vi "tsapp_configure_baudrate_can_win32.vi"(1 "AppName":string, 2 "配置波特率":T1={"硬件类型"=3, "硬件子类型"=5, "ABaudrateKbps"=500.0, "AListenOnly"=enum."Normal", "Int120Ohm"=enum."Disable", "EnableChannel"=enum."Enable", "AHwChannel"=0, "AAppChannel"=0} {"AAppChannel" items=["CHN1", "CHN2", "CHN3", "CHN4", "CHN5", "CHN6", "CHN7", "CHN8", "CHN9", "CHN10", "CHN11", "CHN12", "CHN13", "CHN14", "CHN15", "CHN16", "CHN17", "CHN18", "CHN19", "CHN20", "CHN21", "CHN22", "CHN23", "CHN24", "CHN25", "CHN26", "CHN27", "CHN28", "CHN29", "CHN30", "CHN31", "CHN32"]; "AHwChannel" items=["CHN1", "CHN2", "CHN3", "CHN4", "CHN5", "CHN6", "CHN7", "CHN8", "CHN9", "CHN10", "CHN11", "CHN12", "CHN13", "CHN14", "CHN15", "CHN16", "CHN17", "CHN18", "CHN19", "CHN20", "CHN21", "CHN22", "CHN23", "CHN24", "CHN25", "CHN26", "CHN27", "CHN28", "CHN29", "CHN30", "CHN31", "CHN32"]; "硬件子类型" items=["BUS_UNKNOWN_TYPE", "TSCAN_PRO_4", "TSCAN_LITE_2", "TSCANMini", "TSLinMini", "TSCANFDmini", "TSCAN_LIN_IO_2", "TSCAN_LITE_2", "TSCANLIN", "TSCAN_FD_Mini_1"]; "硬件类型" items=["BUS_UNKNOWN_TYPE", "TS_TCP_DEVICE", "XL_USB_DEVICE", "TS_USB_DEVICE", "PEAK_USB_DEVICE", "KVASER_USB_DEVICE", "ZLG_USB_DEVICE", "ICS_USB_DEVICE", "TS_TC1005_DEVICE"]}, 3 "错误输入（无错误）":errorcluster) -> (9 "InitSts":bool, 10 "错误输出":errorcluster)   [LabVIEW 2016]
uses:
  Ctrl/CAN_BaudInfo.ctl
  TSMaster.dll
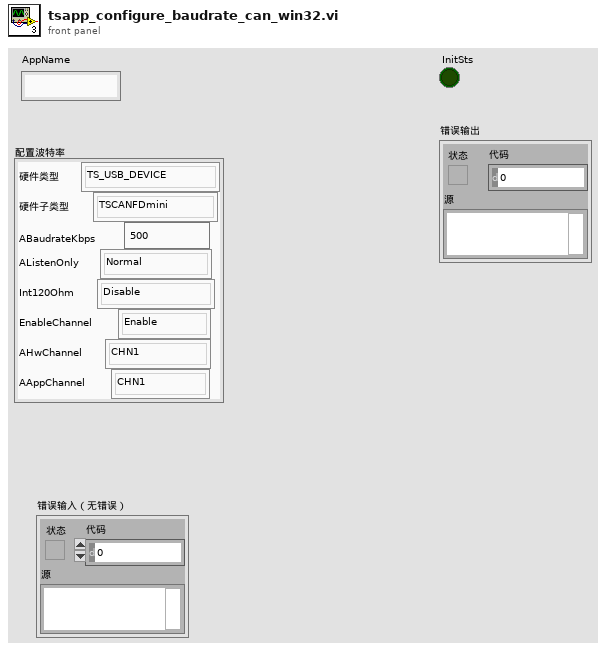
[diagram p1: front panel]
types:
  T1 = typedef "CAN_BaudInfo.ctl" = cluster{"硬件类型":i32, "硬件子类型":i32, "ABaudrateKbps":sgl, "AListenOnly":enum16{"Normal", "ListenOnly"}, "Int120Ohm":enum16{"Disable", "Enable"}, "EnableChannel":enum16{"Disable", "Enable"}, "AHwChannel":i32, "AAppChannel":i32}
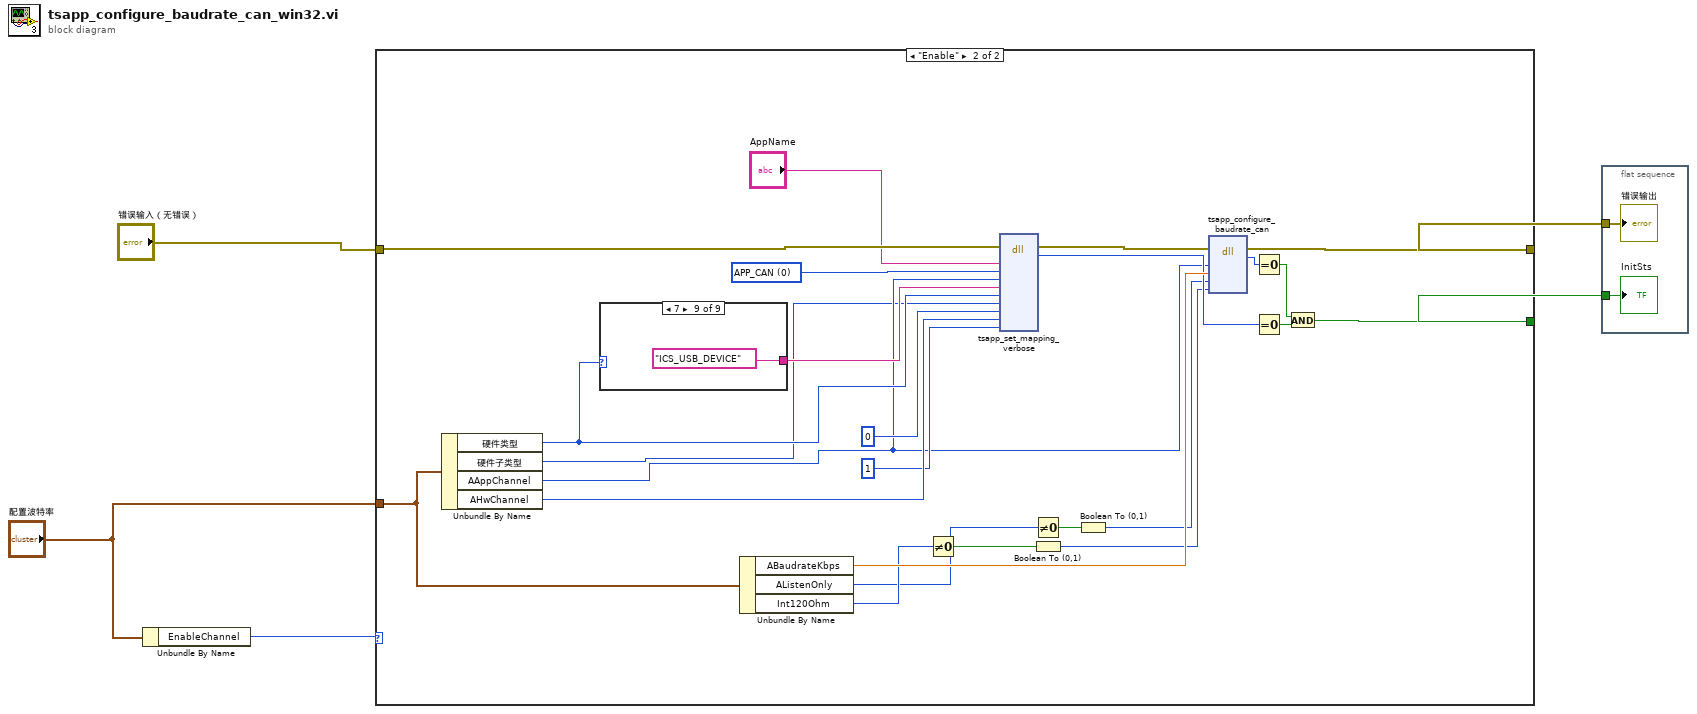
[diagram p0: block diagram]
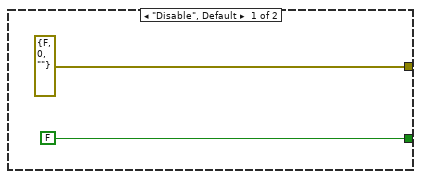
[diagram p2: hidden frame]
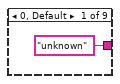
[diagram p3: hidden frame]
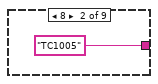
[diagram p4: hidden frame]
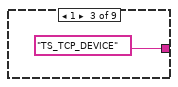
[diagram p5: hidden frame]
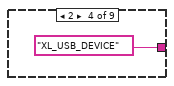
[diagram p6: hidden frame]
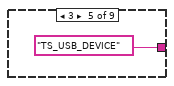
[diagram p7: hidden frame]
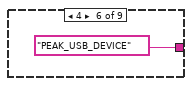
[diagram p8: hidden frame]
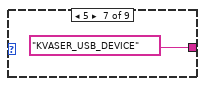
[diagram p9: hidden frame]
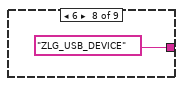
[diagram p10: hidden frame]
diagram:
  n1 = Unbundle By Name("配置波特率") -> ("EnableChannel"=w2:enum16{"Disable", "Enable"})
  n2 = case shown="\"Enable\"" w2 {
    tunnel: "错误输入（无错误）" -> [_ w31]
    tunnel: [errorcluster {"status"=FALSE, "code"=0, "source"=""} ("错误输出") w27] -> w4
    tunnel: [FALSE w14] -> w3
    tunnel: "配置波特率" -> [_ w20]
    frame "Disable", Default {
    }
    frame "Enable" {
      w30 = 0 items=["APP_CAN", "APP_LIN"] ("AAppChannelType")
      n3 = Unbundle By Name(w20) -> ("硬件类型"=w10:i32, "硬件子类型"=w8:i32, "AAppChannel"=w9:i32, "AHwChannel"=w19:i32)
      n4 = case shown="7" w10 {
        tunnel: ["unknown" ("AHardwareName") "TC1005" ("AHardwareName") "TS_TCP_DEVICE" ("AHardwareName") "XL_USB_DEVICE" ("AHardwareName") "TS_USB_DEVICE" ("AHardwareName") "PEAK_USB_DEVICE" ("AHardwareName") "KVASER_USB_DEVICE" ("AHardwareName") "ZLG_USB_DEVICE" ("AHardwareName") "ICS_USB_DEVICE" ("AHardwareName")] -> w29
        frame 0, Default {
        }
        frame 8 {
        }
        frame 1 {
        }
        frame 2 {
        }
        frame 3 {
        }
        frame 4 {
        }
        frame 5 {
        }
        frame 6 {
        }
        frame 7 {
        }
      }
      n5 = Unbundle By Name(w20) -> ("ABaudrateKbps"=w26:sgl, "AListenOnly"=w24:enum16{"Normal", "ListenOnly"}, "Int120Ohm"=w25:enum16{"Disable", "Enable"})
      n6 = Not Equal To 0?(x=w25) -> (x != 0?=w22:bool)
      n7 = dll-call lib="C:/Users/Eric/Desktop/LabVIEW/TSMasterAPI/Win32/CANopen_TS_2015/TSMaster.dll" fn="tsapp_set_mapping_verbose"(error in=w31, "FAppName"="AppName", "AChnType"=w30, "FAppChannelIndex"=w9, "AHWDeviceName"=w29, "AHWDeviceType"=w10, "AHWDeviceSubType"=w8, "AIdxHW"=0 ("AHardwareSubType"), "AIdxHWChn"=w19, "FMappingDisabled"=u32 1) -> (error out=w32:errorcluster, "tsapp_set_channel_mapping"=w17:i32)  [unwired: 11 in, 1 out]
      n8 = Not Equal To 0?(x=w24) -> (x != 0?=w23:bool)
      n9 = Boolean To (0,1)(Boolean=w22) -> (0, 1=w11:i16)
      n10 = Boolean To (0,1)(Boolean=w23) -> (0, 1=w12:i16)
      n11 = dll-call lib="C:/Users/Eric/Desktop/LabVIEW/TSMasterAPI/Win32/CANopen_TS_2015/TSMaster.dll" fn="tsapp_configure_baudrate_can"(error in=w32, "AIdxChn"=w9, "ABaudrateKbps"=w26, "AListenOnly"=w12, "AInstallTermResistor120Ohm"=w11) -> (error out=w27:errorcluster, "tsapp_configure_baudrate_can"=w18:i32)  [unwired: 6 in, 1 out]
      n12 = Equal To 0?(x=w18) -> (x = 0?=w16:bool)
      n13 = Equal To 0?(x=w17) -> (x = 0?=w15:bool)
      n14 = And(x=w16, y=w15) -> (x .and. y?=w14:bool)
    }
  }
  n15 = flat-sequence {
    tunnel: w4 -> [w43]
    tunnel: w3 -> [w42]
    frame #0 {
      "错误输出" <- w43
      "InitSts" <- w42
    }
  }
